vi "tlc_File Module.vi"(7 "Command":T3, 8 "error in (no error)":errorcluster, 9 "Cue Array Input":T1[](array[typedef]) {"Channels"."Intensity" min=0.0 max=100.0 step=1.0 format="%#.0f"}, 10 "Path":path) -> (0 "error out":errorcluster, 1 "Cue Array Output":T1[](array[typedef]) {"Channels"."Intensity" min=0.0 max=100.0 step=1.0 format="%#.0f"})   [LabVIEW 2018]
uses:
  tlc_File_Command Control.ctl
  Controls/tlc_Cue_Information.ctl
  Controls/channel.ctl
panel:
  # "Local Data"
  # "Input Data"
  # "Output Data"
  # "No Local Data"
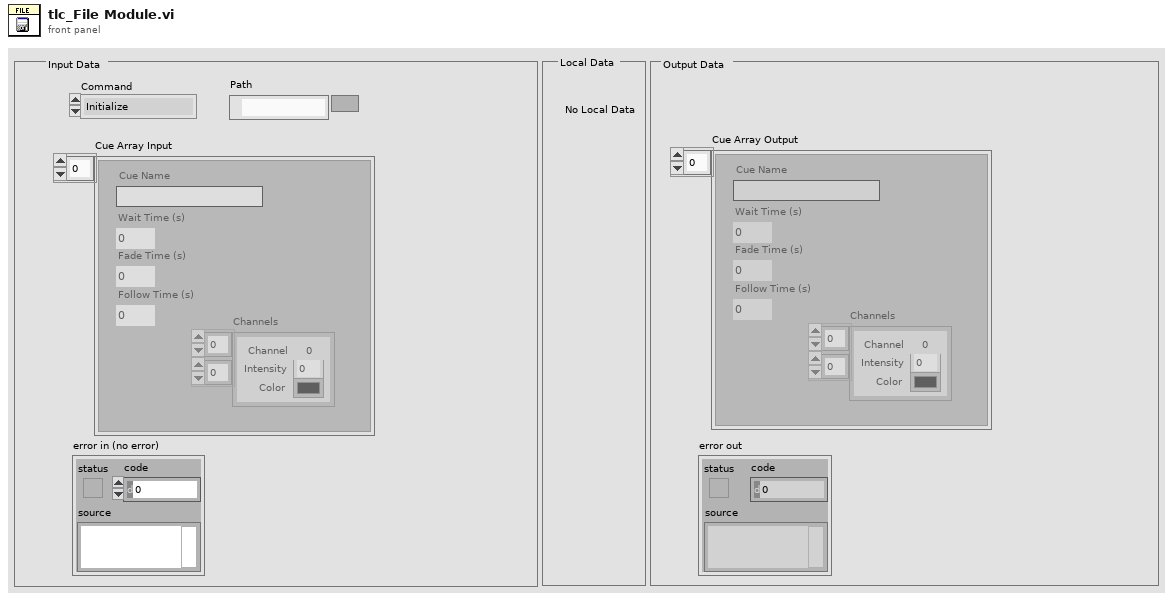
[diagram p1: front panel]
types:
  T1 = typedef "tlc_Cue_Information.ctl" = cluster{"Cue Name":string, "Wait Time (s)":u32, "Fade Time (s)":u32, "Follow Time (s)":u32, "Channels":T2[][]}
  T2 = typedef "channel.ctl" = cluster{"Intensity":dbl, " Color":u32, "Channel":i32}
  T3 = typedef "tlc_File_Command Control.ctl" = enum16{"Initialize", "Save Cues", "Load Cues", "Shutdown"}
  T4 = enum16{"open", "open or create", "create or replace", "create", "open (read only)"}
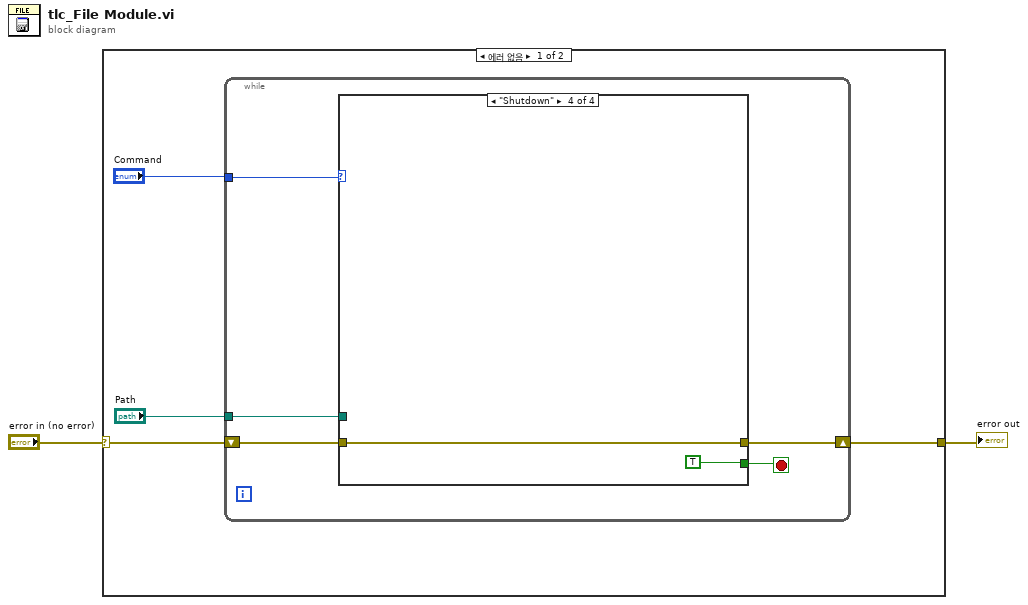
[diagram p0: block diagram]
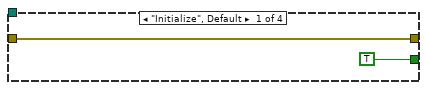
[diagram p2: hidden frame]
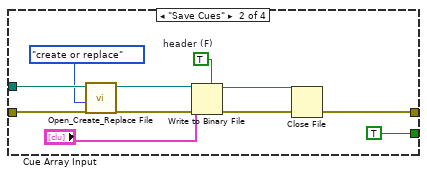
[diagram p3: hidden frame]
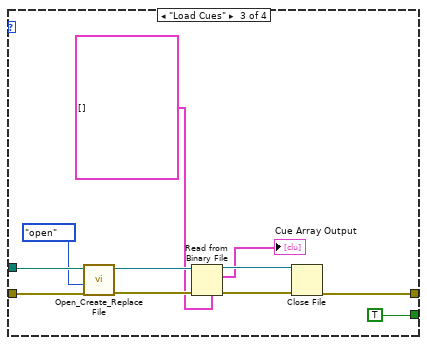
[diagram p4: hidden frame]
diagram:
  n1 = case shown="에러 없음" "error in (no error)" {
    selector: "error in (no error)" -> [w6 w38]
    tunnel: [w5 w38] -> w1
    frame No Error {
      n2 = while {
        shift-right: [w9] -> w5
        shift-left: w6 -> [w10]
        tunnel: "Path" -> [w8]
        tunnel: "Command" -> [w7]
        stop <- w11 stop-if-true
        n3 = case shown="\"Shutdown\"" w7 {
          tunnel: [TRUE TRUE TRUE TRUE] -> w11
          tunnel: w10 -> [w12 w16 w28 w37]
          tunnel: [w12 w15 w27 w37] -> w9
          tunnel: w8 -> [_ w23 w34 _]
          frame "Initialize", Default {
          }
          frame "Save Cues" {
            w17 = TRUE  # header (F)
            n4 = call <vilib>:"Open_Create_Replace File.vi"("error in (no error)"=w16, "function (open:0)"=T4."create or replace", "file path"=w23) -> ("error out"=w18:errorcluster, "refnum"=w21:refnum<file>)  [unwired: 5 in, 2 out]
            n5 = Write to Binary File(file (use dialog)=w21, data="Cue Array Input", error in=w18, 5:w17) -> (refnum out=w20:refnum<file>, error out=w19:errorcluster)  [unwired: 2 in, 1 out]
            n6 = Close File(refnum=w20, error in=w19) -> (error out=w15:errorcluster)  [unwired: 1 out]
          }
          frame "Load Cues" {
            n7 = call <vilib>:"Open_Create_Replace File.vi"("error in (no error)"=w28, "function (open:0)"=T4."open", "file path"=w34) -> ("error out"=w31:errorcluster, "refnum"=w33:refnum<file>)  [unwired: 5 in, 2 out]
            n8 = Read from Binary File(5:T1[] [], 8:w31, 11:w33) -> (0:w30:errorcluster, 2:→"Cue Array Output":T1[], 3:w32:refnum<file>)  [unwired: 3 in, 1 out]
            n9 = Close File(refnum=w32, error in=w30) -> (error out=w27:errorcluster)  [unwired: 1 out]
          }
          frame "Shutdown" {
          }
        }
      }
    }
    frame Error {
    }
  }
  "error out" <- w1
